vi "Keyence.Main.Tune.vi"(8 "error in (no error)":errorcluster, 9 "Timeout_ms":i32, 10 "Bank":u8, 11 "TCP Network Connection in":refnum<k5>) -> (0 "error out":errorcluster, 2 "Tune succeded":bool, 3 "TCP Network Connection out":refnum<k5>)   [LabVIEW 2015]
uses:
  LowLevel/Keyence.Cmd.ParametersBank.ctl
  LowLevel/Keyence.Cmd.OperationCommands.ctl
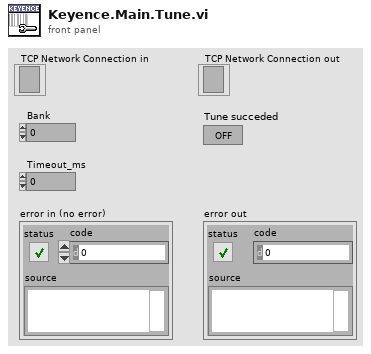
[diagram p1: front panel]
types:
  T1 = typedef "Keyence.Cmd.ParametersBank.ctl" = enum16{"Decoding Area", "Scan.DynamicRange"}
  T2 = typedef "Keyence.Cmd.OperationCommands.ctl" = enum16{"Area limit"}
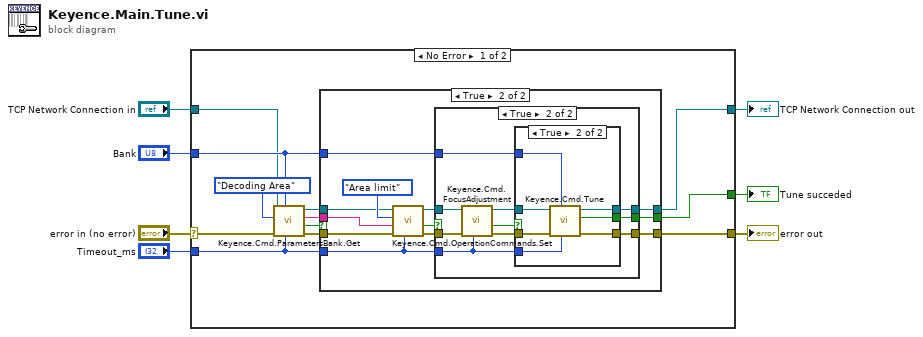
[diagram p0: block diagram]
diagram:
  n1 = case shown="No Error" "error in (no error)" {
    selector: "error in (no error)" -> [w8 w56]
    tunnel: "Timeout_ms" -> [w19 _]
    tunnel: [w18 _] -> w6
    tunnel: "Bank" -> [w17 _]
    tunnel: [w16 w55] -> w4
    tunnel: "TCP Network Connection in" -> [w15 w55]
    tunnel: [w14 w56] -> w2
    frame No Error {
      n2 = call "Keyence.Cmd.ParametersBank.Get.vi"("Timeout [ms] (1000)"=w19, "Bank"=w17, "error in"=w8, "Cmd"=Keyence.Cmd.ParametersBank."Decoding Area", "cID in"=w15) -> ("error out"=w10:errorcluster, "OK?"=w12:bool, "Response"=w11:string, "cID out"=w9:refnum<k5>)  [unwired: 3 in]
      n3 = case shown="True" w12 {
        tunnel: [w20 w33] -> w14
        tunnel: [w21 w32] -> w16
        tunnel: w19 -> [_ w28]
        tunnel: w9 -> [w21 w27]
        tunnel: w10 -> [w20 w26]
        tunnel: w11 -> [_ w25]
        tunnel: w17 -> [_ w23]
        tunnel: [_ w22] -> w18
        frame False {
        }
        frame True {
          n4 = call "Keyence.Cmd.OperationCommands.Set.vi"("Timeout [ms] (1000)"=w28, "error in"=w26, "Parameters"=w25, "Cmd"=Keyence.Cmd.OperationCommands."Area limit", "cID in"=w27) -> ("error out"=w30:errorcluster, "OK?"=w24:bool, "cID out"=w29:refnum<k5>)  [unwired: 3 in, 1 out]
          n5 = case shown="True" w24 {
            tunnel: [w34 w37] -> w33
            tunnel: [w35 w38] -> w32
            tunnel: w30 -> [w34 w45]
            tunnel: w29 -> [w35 w44]
            tunnel: w28 -> [_ w39]
            tunnel: w23 -> [_ w40]
            tunnel: [_ w36] -> w22
            frame False {
            }
            frame True {
              n6 = call "Keyence.Cmd.FocusAdjustment.vi"("Timeout [ms] (1000)"=w39, "error in"=w45, "cID in"=w44) -> ("error out"=w41:errorcluster, "OK?"=w42:bool, "cID out"=w43:refnum<k5>)  [unwired: 5 in, 1 out]
              n7 = case shown="True" w42 {
                tunnel: w43 -> [w47 w54]
                tunnel: w41 -> [w46 w53]
                tunnel: w40 -> [_ w52]
                tunnel: w39 -> [_ w51]
                tunnel: [w47 w50] -> w38
                tunnel: [w46 w49] -> w37
                tunnel: [_ w48] -> w36
                frame False {
                }
                frame True {
                  n8 = call "Keyence.Cmd.Tune.vi"("Timeout [ms] (1000)"=w51, "Bank"=w52, "error in (no error)"=w53, "cID in"=w54) -> ("error out"=w49:errorcluster, "Tune succeded"=w48:bool, "cID out"=w50:refnum<k5>)  [unwired: 4 in, 1 out]
                }
              }
            }
          }
        }
      }
    }
    frame Error {
    }
  }
  "Tune succeded" <- w6
  "TCP Network Connection out" <- w4
  "error out" <- w2
